vi "AlliGator ICCD DAQ Parameters Dialog.vi"(6 "Default Outcome (if Ignore)":bool, 8 "Cancel Button Text":string="Cancel", 9 "OK Button Text":string="OK", 11 "Message":string) -> (0 "OK?":bool, 3 "ICCD Camera Acquisition Parameters out":T1={"V MCP"=1.0, "X Hardware Binning"=0.0, "Y Hardware Binning"=0.0, "Gate Image Integration"=0.0, "Laser Power"=0.0})   [LabVIEW 2021, in "AlliGator Camera Noise Influence on Lifetime.lvlib"]
uses:
  Camera Noise Influence on Lifetime/AlliGator Camera Noise Influence on Lifetime.lvlib
  Files/AlliGator ICCD-specific Information.ctl
  Files/AlliGator Files.lvlib
panel:
  in  "Use Dataset Parameters":bool
  in  "ICCD-specific Information":T1={"V MCP"=1.0, "X Hardware Binning"=0.0, "Y Hardware Binning"=0.0, "Gate Image Integration"=0.0, "Laser Power"=0.0}
  in  "Do not show this dialog again":bool
  in  "Cancel":bool
  in  "OK":bool
  out "Displayed Message":string
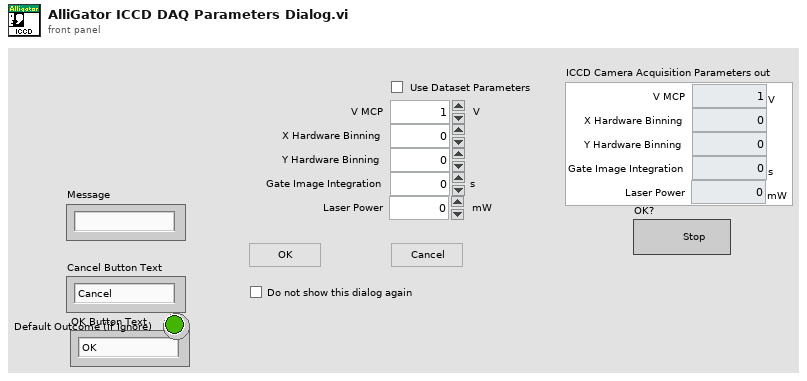
[diagram p1: front panel]
types:
  T1 = typedef "AlliGator Files.lvlib/AlliGator ICCD-specific Information.ctl" = cluster{"V MCP":dbl[unit], "X Hardware Binning":dbl, "Y Hardware Binning":dbl, "Gate Image Integration":dbl[unit], "Laser Power":dbl[unit]}
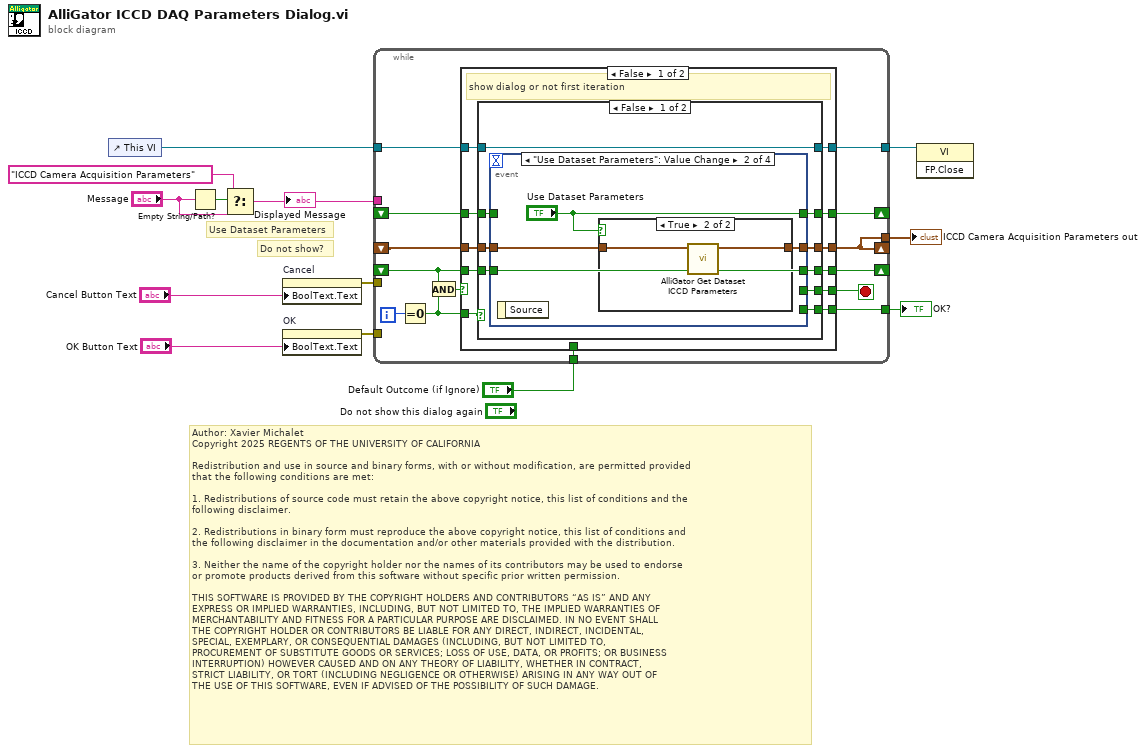
[diagram p0: block diagram]
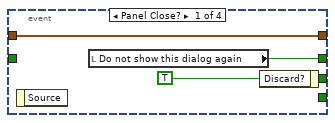
[diagram p2: hidden frame]
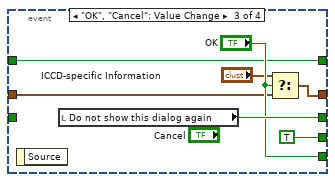
[diagram p4: hidden frame]
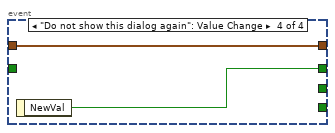
[diagram p5: hidden frame]
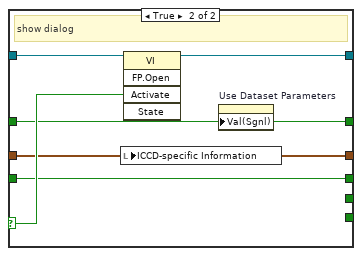
[diagram p6: hidden frame]
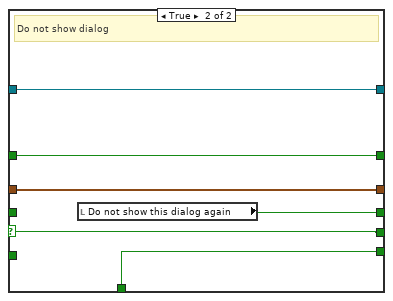
[diagram p7: hidden frame]
diagram:
  # "Author: Xavier Michalet\nCopyright 2025 REGENTS OF THE UNIVERSITY OF CALIFORNIA\n\nRedistribution and use in source and binary forms, with or without modification, are permitted provided\nthat the following conditions are met:\n\n1. Redistributions of source code must retain the above copyright notice, this list of conditions and the\nfollowing disclaimer.\n\n2. Redistributions in binary form must reproduce the above copyright notice, this list of conditions and\nthe following disclaimer in the documentation and/or other materials provided with the distribution.\n\n3. Neither the name of the copyright holder nor the names of its contributors may be used to endorse \nor promote products derived from this software without specific prior written permission.\n\nTHIS SOFTWARE IS PROVIDED BY THE COPYRIGHT HOLDERS AND CONTRIBUTORS “AS IS” AND ANY \nEXPRESS OR IMPLIED WARRANTIES, INCLUDING, BUT NOT LIMITED TO, THE IMPLIED WARRANTIES OF\nMERCHANTABILITY AND FITNESS FOR A PARTICULAR PURPOSE ARE DISCLAIMED. IN NO EVENT SHALL\nTHE COPYRIGHT HOLDER OR CONTRIBUTORS BE LIABLE FOR ANY DIRECT, INDIRECT, INCIDENTAL, \nSPECIAL, EXEMPLARY, OR CONSEQUENTIAL DAMAGES (INCLUDING, BUT NOT LIMITED TO, \nPROCUREMENT OF SUBSTITUTE GOODS OR SERVICES; LOSS OF USE, DATA, OR PROFITS; OR BUSINESS\nINTERRUPTION) HOWEVER CAUSED AND ON ANY THEORY OF LIABILITY, WHETHER IN CONTRACT, \nSTRICT LIABILITY, OR TORT (INCLUDING NEGLIGENCE OR OTHERWISE) ARISING IN ANY WAY OUT OF\nTHE USE OF THIS SOFTWARE, EVEN IF ADVISED OF THE POSSIBILITY OF SUCH DAMAGE."
  # "Use Dataset Parameters"
  # "Do not show?"
  n1 = control-ref of="This VI"() -> (w3:refnum<vi>)
  n2 = Empty String/Path?(string/path="Message") -> (empty?=w5:bool)
  n3 = Select(t="ICCD Camera Acquisition Parameters", s=w5, f="Message") -> (s? t:f=w1:string)
  "Displayed Message" <- w1
  n4 = property on="Cancel" class="Bool"("BoolText.Text"="Cancel Button Text") -> (error out=w10:errorcluster)  [unwired: 2 in, 1 out]
  n5 = property on="OK" class="Bool"("BoolText.Text"="OK Button Text") -> (error out=w9:errorcluster)  [unwired: 2 in, 1 out]
  n6 = while {
    shift-right: [w27] -> _
    shift-left: _ -> [w25]
    tunnel: w3 -> [w21]
    tunnel: [w20] -> w13
    tunnel: w10 -> [_]
    tunnel: w9 -> [_]
    tunnel: [w19] -> w8
    tunnel: "Default Outcome (if Ignore)" -> [w18]
    shift-right: [w16] -> _
    shift-left: _ -> [w17]
    tunnel: [w16] -> w6
    tunnel: w1 -> [_]
    shift-right: [w14] -> _
    shift-left: _ -> [w15]
    i -> [w26]
    stop <- w23 stop-if-true
    n7 = Equal To 0?(x=w26) -> (x = 0?=w22:bool)
    n8 = And(x=w25, y=w22) -> (x .and. y?=w24:bool)
    n9 = case shown="False" w24 {
      selector: w24 -> [_ w78]
      tunnel: [w38 w78] -> w23
      tunnel: [w37 w76] -> w27
      tunnel: w25 -> [w36 _]
      tunnel: w22 -> [w35 _]
      tunnel: w21 -> [w34 w77]
      tunnel: [w33 w77] -> w20
      tunnel: [w32 w75] -> w19
      tunnel: w18 -> [_ w75]
      tunnel: w17 -> [w31 w74]
      tunnel: [w30 w74] -> w16
      tunnel: w15 -> [w29 w73]
      tunnel: [w28 w73] -> w14
      frame False {
        # "show dialog or not first iteration"
        n10 = case shown="False" w35 {
          selector: w35 -> [_ w71]
          tunnel: [w47 _] -> w38
          tunnel: [w46 w69] -> w37
          tunnel: w36 -> [w45 w69]
          tunnel: w34 -> [w44 w72]
          tunnel: [w44 w70] -> w33
          tunnel: [w43 _] -> w32
          tunnel: w31 -> [w42 w68]
          tunnel: [w41 w68] -> w30
          tunnel: w29 -> [w40 w67]
          tunnel: [w39 w67] -> w28
          frame False {
            n11 = event shown="[1] \"Use Dataset Parameters\": Value Change" {
              selector: _ -> [_ _ _ _]
              dyn-events: _ -> [_ _ _ _]
              timeout: _ -> [_ _ _ _]
              tunnel: [w50 _ TRUE ("Discard?") _] -> w47
              tunnel: [w49 w54 w63 w66] -> w46
              tunnel: w45 -> [_ w54 _ _]
              tunnel: [_ _ "OK" _] -> w43
              tunnel: w42 -> [w48 w52 w60 w65]
              tunnel: [w48 w51 w59 w65] -> w41
              tunnel: [_ "Use Dataset Parameters" w58 _] -> w39
              tunnel: w40 -> [_ _ w58 _]
              event Panel Close? {
                w50 = TRUE ("Discard?")
                n12 = event-data() -> ()  [unwired: 1 in, 1 out]
                n13 = local read "Do not show this dialog again"() -> (w49:bool)
                n14 = event-data("Discard?"=w50) -> ()  [unwired: 1 in, 1 out]
              }
              event "Use Dataset Parameters": Value Change {
                n15 = event-data() -> ()  [unwired: 1 in, 1 out]
                n16 = case shown="True" "Use Dataset Parameters" {
                  tunnel: w52 -> [w55 w57]
                  tunnel: [w55 w56] -> w51
                  frame False {
                  }
                  frame True {
                    n17 = call "AlliGator Get Dataset ICCD Parameters.vi"("ICCD Camera Acquisition Parameters in"=w57) -> ("ICCD Camera Acquisition Parameters out"=w56:T1)  [unwired: 9 in, 1 out]
                  }
                }
              }
              event "OK", "Cancel": Value Change {
                n18 = event-data() -> ()  [unwired: 1 in, 1 out]
                n19 = local read "Do not show this dialog again"() -> (w63:bool)
                n20 = Select(t="ICCD-specific Information", s="OK", f=w60) -> (s? t:f=w59:T1)
              }
              event "Do not show this dialog again": Value Change {
                n21 = event-data() -> ("NewVal"=w66:bool)  [unwired: 1 in]
              }
            }
          }
          frame True {
            # "show dialog"
            n22 = local write "ICCD-specific Information"(w68) -> ()
            n23 = invoke class="VI" method="FP.Open"(reference=w72, "Activate"=w71) -> (reference out=w70:refnum<vi>)  [unwired: 3 in, 4 out]
            n24 = property on="Use Dataset Parameters" class="Bool (strict)"("Val(Sgnl)"=w67) -> ()  [unwired: 2 in, 2 out]
          }
        }
      }
      frame True {
        # "Do not show dialog"
        n25 = local read "Do not show this dialog again"() -> (w76:bool)
      }
    }
  }
  "OK?" <- w8
  "ICCD Camera Acquisition Parameters out" <- w6
  n26 = invoke class="VI" method="FP.Close"(reference=w13) -> ()  [unwired: 2 in, 3 out]
